vi "Tank height state.vi"(7 "Set state:":bool, 8 "Tank height":dbl, 9 "Tank Valves":T1=enum."Tank B", 10 "Tank name":string) -> (0 "State":bool)   [LabVIEW 2011]
uses:
  Tank Valves.ctl
  Valve_Pump.ctl
  Pumps_Valves_Dependencies_Global.vi
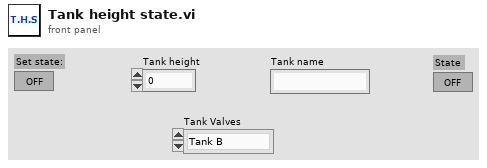
[diagram p1: front panel]
types:
  T1 = typedef "Tank Valves.ctl" = enum16{"Salt Saturator", "Tank A", "Tank B", "Tank C", "Tank D"}
  T2 = typedef "Valve_Pump.ctl" = enum16{"Main Rack Power", "Pump Power", "Valve Power", "V4", "V5", "V6", "V7", "V8", "V9", "V10", "V11", "V12", "V13", "V14", "V15", "V18", "V19", "V20", "V21", "V22", "V23", "V24", "V25", "V26", "V27", "V28", "V29", "V30", "V31", "V32", "V33", "V34", "Pump A", "Pump B", "Pump C", "Pump D"}
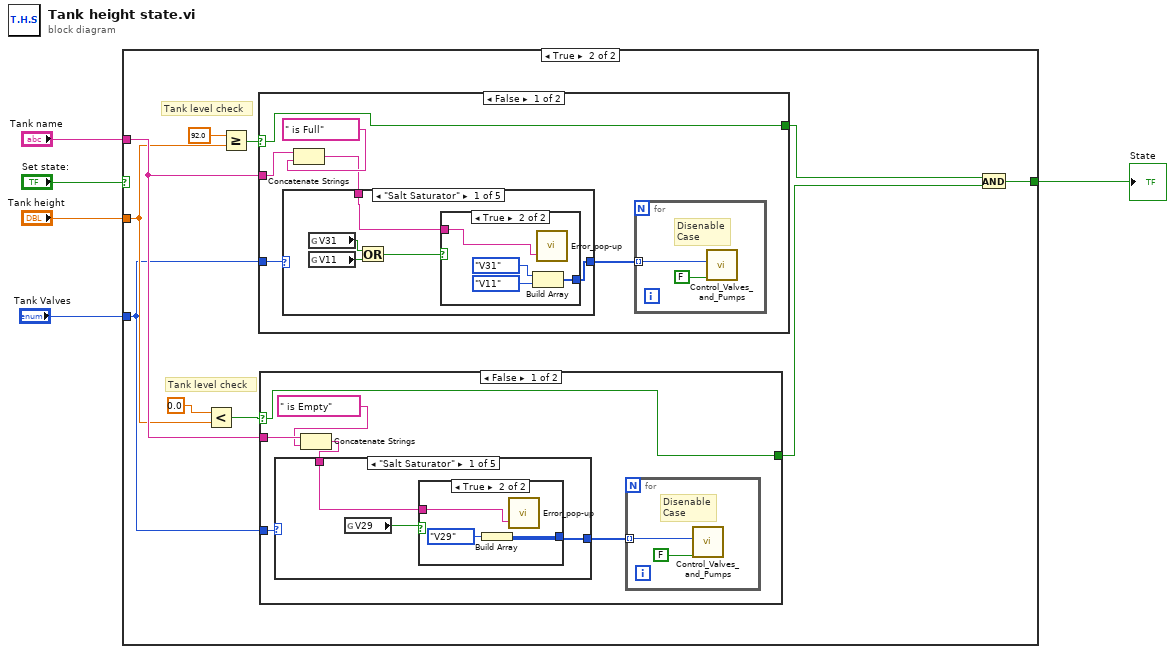
[diagram p0: block diagram]
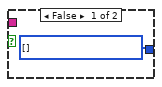
[diagram p3: hidden frame]
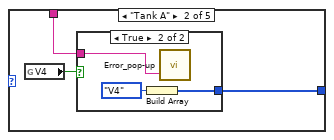
[diagram p4: hidden frame]
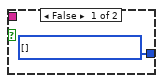
[diagram p5: hidden frame]
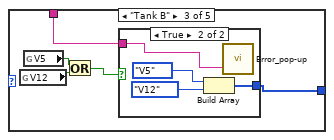
[diagram p6: hidden frame]
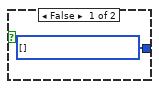
[diagram p7: hidden frame]
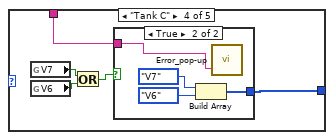
[diagram p8: hidden frame]
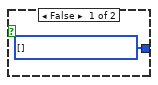
[diagram p9: hidden frame]
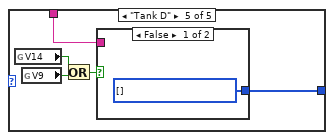
[diagram p10: hidden frame]
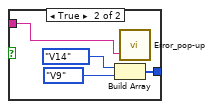
[diagram p11: hidden frame]
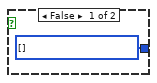
[diagram p13: hidden frame]
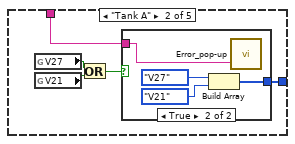
[diagram p14: hidden frame]
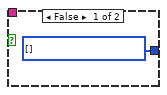
[diagram p15: hidden frame]
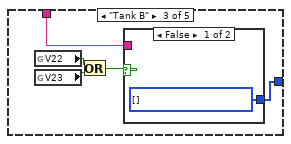
[diagram p16: hidden frame]
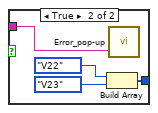
[diagram p17: hidden frame]
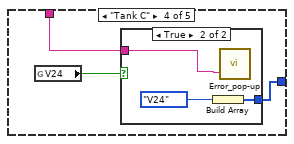
[diagram p18: hidden frame]
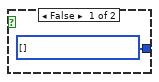
[diagram p19: hidden frame]
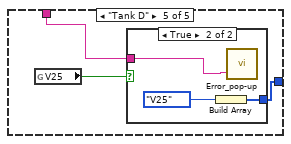
[diagram p20: hidden frame]
diagram:
  n1 = case shown="True" "Set state:" {
    selector: "Set state:" -> [w6 _]
    tunnel: "Tank name" -> [_ w12]
    tunnel: "Tank height" -> [_ w11]
    tunnel: [w6 w8] -> w1
    tunnel: "Tank Valves" -> [_ w7]
    frame False {
    }
    frame True {
      # "Tank level check"
      # "Tank level check"
      n2 = Less?(x=0.0, y=w11) -> (x < y?=w13:bool)
      n3 = Greater Or Equal?(x=92.0, y=w11) -> (x >= y?=w14:bool)
      n4 = case shown="False" w14 {
        selector: w14 -> [w73 w122]
        tunnel: [w73 w122] -> w9
        tunnel: w12 -> [w74 _]
        tunnel: w7 -> [w72 _]
        frame False {
          n5 = Concatenate Strings(w74, " is Full") -> (w71:string)
          n6 = case shown="\"Salt Saturator\"" w72 {
            tunnel: [w82 w92 w102 w110 w117] -> w70
            tunnel: w71 -> [w78 w88 w98 w109 w116]
            frame "Salt Saturator" {
              n7 = global read "Pumps_Valves_Dependencies_Global.vi" "V31"() -> (w81:bool)
              n8 = global read "Pumps_Valves_Dependencies_Global.vi" "V11"() -> (w80:bool)
              n9 = Or(x=w81, y=w80) -> (x .or. y?=w79:bool)
              n10 = case shown="True" w79 {
                tunnel: [w83 w86] -> w82
                tunnel: w78 -> [_ w84]
                frame False {
                  w83 = T2[] [] items=["Main Rack Power", "Pump Power", "Valve Power", "V4", "V5", "V6", "V7", "V8", "V9", "V10", "V11", "V12", "V13", "V14", "V15", "V18", "V19", "V20", "V21", "V22", "V23", "V24", "V25", "V26", "V27", "V28", "V29", "V30", "V31", "V32", "V33", "V34", "Pump A", "Pump B", "Pump C", "Pump D"]
                }
                frame True {
                  n11 = Build Array(Valve_Pump."V31" ("Device"), Valve_Pump."V11" ("Device")) -> (w86:T2[])
                  n12 = call "Error_pop-up.vi"("New msg"=w84) -> ()  [unwired: 2 in]
                }
              }
            }
            frame "Tank A" {
              n13 = global read "Pumps_Valves_Dependencies_Global.vi" "V27"() -> (w90:bool)
              n14 = global read "Pumps_Valves_Dependencies_Global.vi" "V21"() -> (w91:bool)
              n15 = Or(x=w90, y=w91) -> (x .or. y?=w89:bool)
              n16 = case shown="True" w89 {
                tunnel: [w93 w95] -> w92
                tunnel: w88 -> [_ w94]
                frame False {
                  w93 = T2[] [] items=["Main Rack Power", "Pump Power", "Valve Power", "V4", "V5", "V6", "V7", "V8", "V9", "V10", "V11", "V12", "V13", "V14", "V15", "V18", "V19", "V20", "V21", "V22", "V23", "V24", "V25", "V26", "V27", "V28", "V29", "V30", "V31", "V32", "V33", "V34", "Pump A", "Pump B", "Pump C", "Pump D"]
                }
                frame True {
                  n17 = Build Array(Valve_Pump."V27" ("Device"), Valve_Pump."V21" ("Device")) -> (w95:T2[])
                  n18 = call "Error_pop-up.vi"("New msg"=w94) -> ()  [unwired: 2 in]
                }
              }
            }
            frame "Tank B" {
              n19 = global read "Pumps_Valves_Dependencies_Global.vi" "V22"() -> (w100:bool)
              n20 = global read "Pumps_Valves_Dependencies_Global.vi" "V23"() -> (w101:bool)
              n21 = Or(x=w100, y=w101) -> (x .or. y?=w99:bool)
              n22 = case shown="False" w99 {
                tunnel: [w103 w105] -> w102
                tunnel: w98 -> [_ w104]
                frame False {
                  w103 = T2[] [] items=["Main Rack Power", "Pump Power", "Valve Power", "V4", "V5", "V6", "V7", "V8", "V9", "V10", "V11", "V12", "V13", "V14", "V15", "V18", "V19", "V20", "V21", "V22", "V23", "V24", "V25", "V26", "V27", "V28", "V29", "V30", "V31", "V32", "V33", "V34", "Pump A", "Pump B", "Pump C", "Pump D"]
                }
                frame True {
                  n23 = Build Array(Valve_Pump."V22" ("Device"), Valve_Pump."V23" ("Device")) -> (w105:T2[])
                  n24 = call "Error_pop-up.vi"("New msg"=w104) -> ()  [unwired: 2 in]
                }
              }
            }
            frame "Tank C" {
              n25 = global read "Pumps_Valves_Dependencies_Global.vi" "V24"() -> (w108:bool)
              n26 = case shown="True" w108 {
                tunnel: [w111 w113] -> w110
                tunnel: w109 -> [_ w112]
                frame False {
                  w111 = T2[] [] items=["Main Rack Power", "Pump Power", "Valve Power", "V4", "V5", "V6", "V7", "V8", "V9", "V10", "V11", "V12", "V13", "V14", "V15", "V18", "V19", "V20", "V21", "V22", "V23", "V24", "V25", "V26", "V27", "V28", "V29", "V30", "V31", "V32", "V33", "V34", "Pump A", "Pump B", "Pump C", "Pump D"]
                }
                frame True {
                  n27 = Build Array(Valve_Pump."V24" ("Device")) -> (w113:T2[])
                  n28 = call "Error_pop-up.vi"("New msg"=w112) -> ()  [unwired: 2 in]
                }
              }
            }
            frame "Tank D" {
              n29 = global read "Pumps_Valves_Dependencies_Global.vi" "V25"() -> (w115:bool)
              n30 = case shown="True" w115 {
                tunnel: [w118 w120] -> w117
                tunnel: w116 -> [_ w119]
                frame False {
                  w118 = T2[] [] items=["Main Rack Power", "Pump Power", "Valve Power", "V4", "V5", "V6", "V7", "V8", "V9", "V10", "V11", "V12", "V13", "V14", "V15", "V18", "V19", "V20", "V21", "V22", "V23", "V24", "V25", "V26", "V27", "V28", "V29", "V30", "V31", "V32", "V33", "V34", "Pump A", "Pump B", "Pump C", "Pump D"]
                }
                frame True {
                  n31 = Build Array(Valve_Pump."V25" ("Device")) -> (w120:T2[])
                  n32 = call "Error_pop-up.vi"("New msg"=w119) -> ()  [unwired: 2 in]
                }
              }
            }
          }
          n33 = for {
            tunnel: w70 -> [w77] mode=indexing
            # "Disenable\nCase"
            n34 = call "Control_Valves_and_Pumps.vi"("Set state:"=FALSE, "Device"=w77) -> ()  [unwired: 10 in]
          }
        }
        frame True {
        }
      }
      n35 = case shown="False" w13 {
        selector: w13 -> [w19 w69]
        tunnel: [w19 w69] -> w10
        tunnel: w12 -> [w22 _]
        tunnel: w7 -> [w18 _]
        frame False {
          n36 = Concatenate Strings(w22, " is Empty") -> (w17:string)
          n37 = case shown="\"Salt Saturator\"" w18 {
            tunnel: [w27 w34 w43 w53 w63] -> w20
            tunnel: w17 -> [w25 w32 w39 w52 w59]
            frame "Salt Saturator" {
              n38 = global read "Pumps_Valves_Dependencies_Global.vi" "V29"() -> (w26:bool)
              n39 = case shown="True" w26 {
                tunnel: [w28 w31] -> w27
                tunnel: w25 -> [_ w29]
                frame False {
                  w28 = T2[] [] items=["Main Rack Power", "Pump Power", "Valve Power", "V4", "V5", "V6", "V7", "V8", "V9", "V10", "V11", "V12", "V13", "V14", "V15", "V18", "V19", "V20", "V21", "V22", "V23", "V24", "V25", "V26", "V27", "V28", "V29", "V30", "V31", "V32", "V33", "V34", "Pump A", "Pump B", "Pump C", "Pump D"]
                }
                frame True {
                  n40 = Build Array(Valve_Pump."V29" ("Device")) -> (w31:T2[])
                  n41 = call "Error_pop-up.vi"("New msg"=w29) -> ()  [unwired: 2 in]
                }
              }
            }
            frame "Tank A" {
              n42 = global read "Pumps_Valves_Dependencies_Global.vi" "V4"() -> (w33:bool)
              n43 = case shown="True" w33 {
                tunnel: [w35 w38] -> w34
                tunnel: w32 -> [_ w36]
                frame False {
                  w35 = T2[] [] items=["Main Rack Power", "Pump Power", "Valve Power", "V4", "V5", "V6", "V7", "V8", "V9", "V10", "V11", "V12", "V13", "V14", "V15", "V18", "V19", "V20", "V21", "V22", "V23", "V24", "V25", "V26", "V27", "V28", "V29", "V30", "V31", "V32", "V33", "V34", "Pump A", "Pump B", "Pump C", "Pump D"]
                }
                frame True {
                  n44 = Build Array(Valve_Pump."V4" ("Device")) -> (w38:T2[])
                  n45 = call "Error_pop-up.vi"("New msg"=w36) -> ()  [unwired: 2 in]
                }
              }
            }
            frame "Tank B" {
              n46 = global read "Pumps_Valves_Dependencies_Global.vi" "V12"() -> (w42:bool)
              n47 = global read "Pumps_Valves_Dependencies_Global.vi" "V5"() -> (w41:bool)
              n48 = Or(x=w41, y=w42) -> (x .or. y?=w40:bool)
              n49 = case shown="True" w40 {
                tunnel: [w44 w46] -> w43
                tunnel: w39 -> [_ w45]
                frame False {
                  w44 = T2[] [] items=["Main Rack Power", "Pump Power", "Valve Power", "V4", "V5", "V6", "V7", "V8", "V9", "V10", "V11", "V12", "V13", "V14", "V15", "V18", "V19", "V20", "V21", "V22", "V23", "V24", "V25", "V26", "V27", "V28", "V29", "V30", "V31", "V32", "V33", "V34", "Pump A", "Pump B", "Pump C", "Pump D"]
                }
                frame True {
                  n50 = Build Array(Valve_Pump."V5" ("Device"), Valve_Pump."V12" ("Device")) -> (w46:T2[])
                  n51 = call "Error_pop-up.vi"("New msg"=w45) -> ()  [unwired: 2 in]
                }
              }
            }
            frame "Tank C" {
              n52 = global read "Pumps_Valves_Dependencies_Global.vi" "V7"() -> (w49:bool)
              n53 = global read "Pumps_Valves_Dependencies_Global.vi" "V6"() -> (w50:bool)
              n54 = Or(x=w49, y=w50) -> (x .or. y?=w51:bool)
              n55 = case shown="True" w51 {
                tunnel: [w54 w56] -> w53
                tunnel: w52 -> [_ w55]
                frame False {
                  w54 = T2[] [] items=["Main Rack Power", "Pump Power", "Valve Power", "V4", "V5", "V6", "V7", "V8", "V9", "V10", "V11", "V12", "V13", "V14", "V15", "V18", "V19", "V20", "V21", "V22", "V23", "V24", "V25", "V26", "V27", "V28", "V29", "V30", "V31", "V32", "V33", "V34", "Pump A", "Pump B", "Pump C", "Pump D"]
                }
                frame True {
                  n56 = Build Array(Valve_Pump."V7" ("Device"), Valve_Pump."V6" ("Device")) -> (w56:T2[])
                  n57 = call "Error_pop-up.vi"("New msg"=w55) -> ()  [unwired: 2 in]
                }
              }
            }
            frame "Tank D" {
              n58 = global read "Pumps_Valves_Dependencies_Global.vi" "V14"() -> (w60:bool)
              n59 = global read "Pumps_Valves_Dependencies_Global.vi" "V9"() -> (w61:bool)
              n60 = Or(x=w60, y=w61) -> (x .or. y?=w62:bool)
              n61 = case shown="False" w62 {
                tunnel: [w64 w66] -> w63
                tunnel: w59 -> [_ w65]
                frame False {
                  w64 = T2[] [] items=["Main Rack Power", "Pump Power", "Valve Power", "V4", "V5", "V6", "V7", "V8", "V9", "V10", "V11", "V12", "V13", "V14", "V15", "V18", "V19", "V20", "V21", "V22", "V23", "V24", "V25", "V26", "V27", "V28", "V29", "V30", "V31", "V32", "V33", "V34", "Pump A", "Pump B", "Pump C", "Pump D"]
                }
                frame True {
                  n62 = Build Array(Valve_Pump."V14" ("Device"), Valve_Pump."V9" ("Device")) -> (w66:T2[])
                  n63 = call "Error_pop-up.vi"("New msg"=w65) -> ()  [unwired: 2 in]
                }
              }
            }
          }
          n64 = for {
            tunnel: w20 -> [w24] mode=indexing
            # "Disenable\nCase"
            n65 = call "Control_Valves_and_Pumps.vi"("Set state:"=FALSE, "Device"=w24) -> ()  [unwired: 10 in]
          }
        }
        frame True {
        }
      }
      n66 = And(x=w9, y=w10) -> (x .and. y?=w8:bool)
    }
  }
  "State" <- w1
